vi "LH6HDGetResponse.vi"(8 "error in (no error)":errorcluster, 11 "TCP Network Connection in":refnum<k5>) -> (0 "error out":errorcluster, 2 "Response":string[](array[string]), 3 "TCP Network Connection out":refnum<k5>)   [LabVIEW 2015]
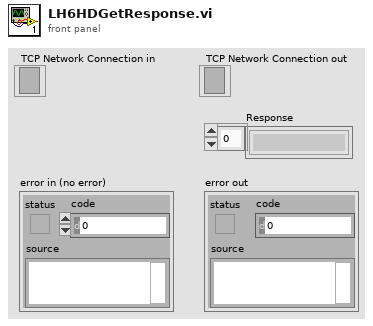
[diagram p1: front panel]
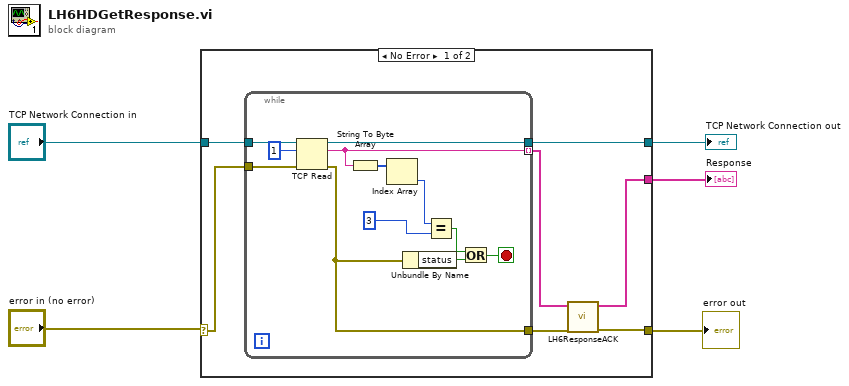
[diagram p0: block diagram]
diagram:
  n1 = case shown="No Error" "error in (no error)" {
    selector: "error in (no error)" -> [w11 w26]
    tunnel: "TCP Network Connection in" -> [w12 w25]
    tunnel: [w7 w26] -> w5
    tunnel: [w8 w25] -> w4
    tunnel: [w6 _] -> w1
    frame No Error {
      n2 = while {
        tunnel: w12 -> [w24]
        tunnel: [w22] -> w10 mode=indexing
        tunnel: w11 -> [w16]
        tunnel: [w15] -> w9
        tunnel: [w14] -> w8
        stop <- w19 stop-if-true
        n3 = TCP Read(connection ID=w24, bytes to read=1, error in (no error)=w16) -> (connection ID out=w14:refnum<k5>, data out=w22:string, error out=w15:errorcluster)  [unwired: 2 in]
        n4 = String To Byte Array(string=w22) -> (unsigned byte array=w18:u8[])
        n5 = Index Array(array=w18) -> (element=w17:u8)  [unwired: 1 in]
        n6 = Unbundle By Name(w15) -> ("status"=w13:bool)
        n7 = Equal?(x=w17, y=u8 3) -> (x = y?=w20:bool)
        n8 = Or(x=w20, y=w13) -> (x .or. y?=w19:bool)
      }
      n9 = call "LH6ResponseACK.vi"("error in"=w9, "Response in"=w10) -> ("error out"=w7:errorcluster, "Response  out"=w6:string[])  [unwired: 8 in]
    }
    frame Error {
    }
  }
  "error out" <- w5
  "Response" <- w1
  "TCP Network Connection out" <- w4
